vi "Global Z-stack acquistion finished flag.vi"() -> ()   [LabVIEW 2020]
panel:
  out "Z-stack acquisition finished flag":bool
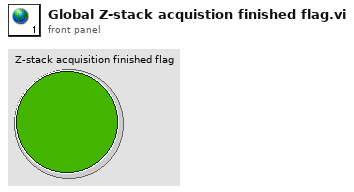
[diagram p1: front panel]
diagram:
